vi "Image Browser Mod.vi"() -> ()   [LabVIEW 2016]
doc: "This example shows how to set up an image browser. An image browser is a concise representation of the images in your database represented as thumbnails on a page. You can use the Browser VIs in NI Vision to configure a browser, configure the selection of one or many images, add new images and remove images to and from a browser, replace an image, and get or set the selection status of an image."
uses:
  <vilib>/vision/NI_Vision_Development_Module.lvlib
panel:
  in  "Image folder":path=path "\\\\eden\\NHMFLDATA/Reference/Pressure/caliphotos/2018_04_12"
  out "Image":T1(plugin-control)
  in  "Stop":bool
  # "Overview: Demonstrates how to use the IMAQ Browser functions to display multiple thumbnail images in a single display. and allow the user to select images from the browser.\nRequirements: Vision Development Software.\nInstructions:\n1. Run the VI.\n2. Click on the images to select or unselect them."
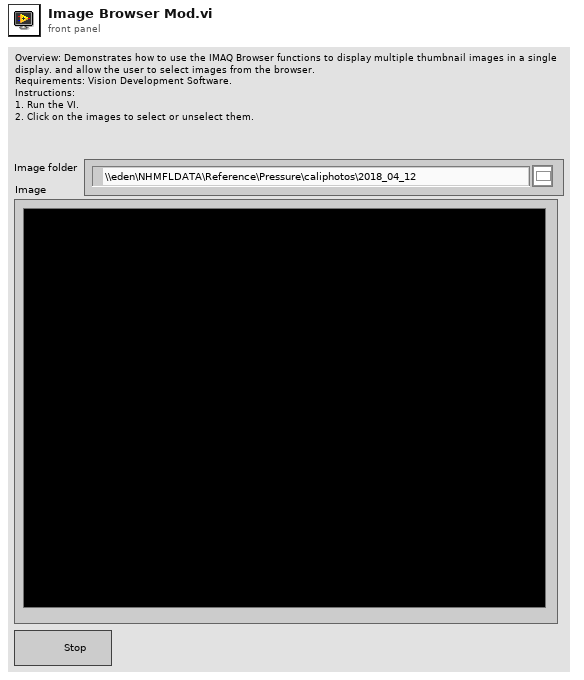
[diagram p1: front panel]
types:
  T1 = typedef "IMAQ Image.ctl" = refnum<image>
  T2 = cluster{"Browser Size":cluster{"X":i32, "Y":i32}, "Images per Line":i32, "Background Color":u32, "Frame Size":i32, "Frame Style":u16}
  T3 = typedef "Image Type" = u32
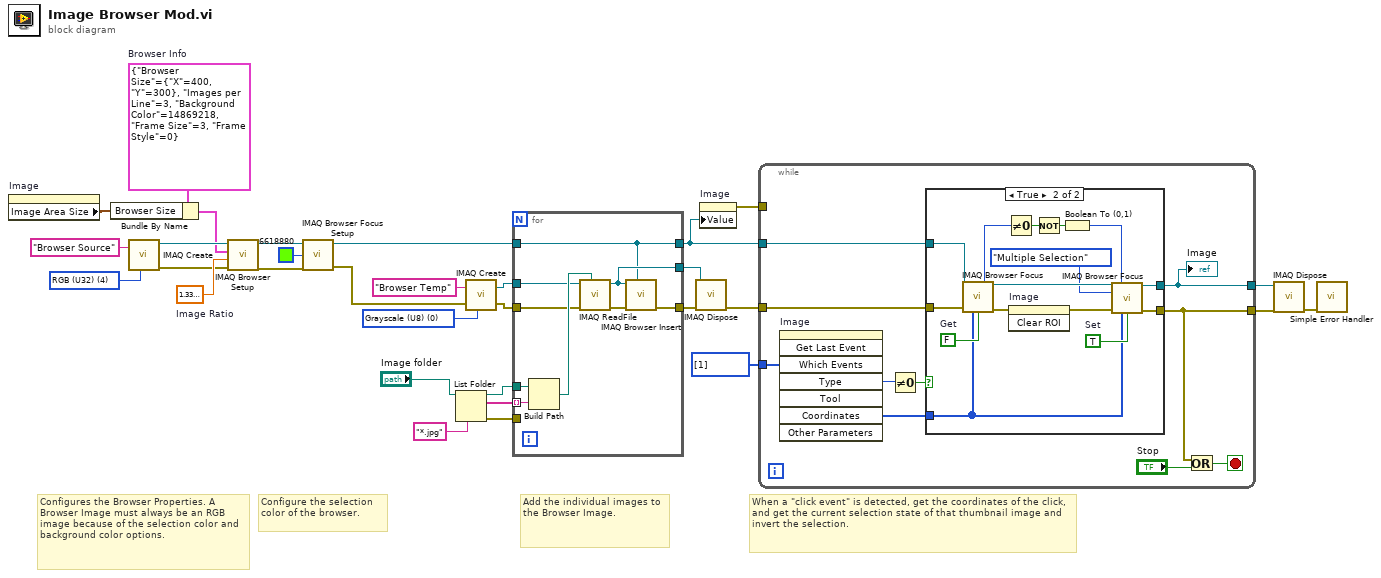
[diagram p0: block diagram]
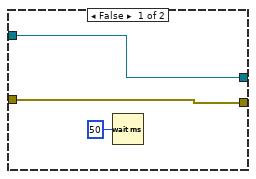
[diagram p2: hidden frame]
diagram:
  w18 = i32[] [1] items=["No Event"=0, "Click Event"=1, "Draw Event"=2, "Size Event"=4, "Scroll Event"=5, "Double Click Event"=8] ("Which Events")
  w31 = sgl 1.33  # Image Ratio
  w6 = T2 {"Browser Size"={"X"=400, "Y"=300}, "Images per Line"=3, "Background Color"=14869218, "Frame Size"=3, "Frame Style"=0}  # Browser Info
  w22 = T3 0 items=["Grayscale (U8)", "Grayscale (I16)", "Grayscale (SGL)", "Complex (CSG)", "RGB (U32)", "HSL (U32)", "RGB (U64)", "Grayscale (U16)"] ("Image Type")
  w24 = T3 4 items=["Grayscale (U8)", "Grayscale (I16)", "Grayscale (SGL)", "Complex (CSG)", "RGB (U32)", "HSL (U32)", "RGB (U64)", "Grayscale (U16)"] ("Image Type")
  # "When a \"click event\" is detected, get the coordinates of the click, and get the current selection state of that thumbnail image and invert the selection."
  # "Add the individual images to the Browser Image."
  # "Configure the selection color of the browser."
  # "Configures the Browser Properties. A Browser Image must always be an RGB image because of the selection color and background color options."
  n1 = property on="Image" class="ImageControl"() -> ("Image Area Size"=w5:cluster{"Width":u32, "Height":u32})  [unwired: 2 in, 2 out]
  n2 = Bundle By Name(cluster=w6, "Browser Size"=w5) -> (w4:T2)
  n3 = call "IMAQ Create"("Image Name"="Browser Source", "Image Type"=w24) -> ("New Image"=w26:T1, "error out"=w25:errorcluster)  [unwired: 3 in]
  n4 = call "IMAQ Browser Setup"("error in (no error)"=w25, "Image Ratio"=w31, "Browser Info"=w4, "Image In"=w26) -> ("error out"=w10:errorcluster, "Image Browser Out"=w11:T1)  [unwired: 2 out]
  n5 = call "IMAQ Browser Focus Setup"("error in (no error)"=w10, "Focus Color"=u32 6618880, "Image Browser In"=w11) -> ("error out"=w8:errorcluster, "Image Browser Out"=w9:T1)  [unwired: 1 in]
  n6 = List Folder(path="Image folder", pattern="*.jpg") -> (path out=w28:path, filenames=w27:string[], error out=w2:errorcluster)  [unwired: 2 in, 1 out]
  n7 = call "IMAQ Create"("Image Name"="Browser Temp", "Image Type"=w22, "error in (no error)"=w8) -> ("New Image"=w14:T1, "error out"=w30:errorcluster)  [unwired: 2 in]
  n8 = for {
    tunnel: w9 -> [w32]
    tunnel: w28 -> [w40]
    tunnel: w27 -> [w37] mode=indexing
    tunnel: w30 -> [w36]
    tunnel: [w35] -> w29
    tunnel: [w32] -> w19
    tunnel: w14 -> [w34]
    tunnel: [w33] -> w13
    tunnel: w2 -> [_]
    n9 = Build Path(base path=w40, name or relative path=w37) -> (appended path=w39:path)
    n10 = call "IMAQ ReadFile"("File Path"=w39, "error in (no error)"=w36, "Image"=w34) -> ("error out"=w38:errorcluster, "Image Out"=w33:T1)  [unwired: 4 in, 3 out]
    n11 = call "IMAQ Browser Insert"("Image Browser In"=w32, "error in (no error)"=w38, "Image to Add"=w33) -> ("error out"=w35:errorcluster)  [unwired: 4 in, 4 out]
  }
  n12 = call "IMAQ Dispose"("Image"=w13, "error in (no error)"=w29) -> ("error out"=w20:errorcluster)  [unwired: 4 in]
  n13 = property on="Image" class="ImageControl"("Value"=w19) -> (error out=w3:errorcluster)  [unwired: 2 in, 1 out]
  n14 = while {
    tunnel: w19 -> [w50]
    tunnel: w20 -> [w47]
    tunnel: w18 -> [w48]
    tunnel: [w45] -> w17
    tunnel: [w42] -> w16
    tunnel: w3 -> [_]
    stop <- w43 stop-if-true
    n15 = invoke on="Image" class="ImageControl" method="Get Last Event"("Which Events"=w48) -> ("Type"=w41:i32, "Coordinates"=w49:i32[])  [unwired: 7 in, 6 out]
    n16 = Not Equal To 0?(x=w41) -> (x != 0?=w46:bool)
    n17 = case shown="True" w46 {
      tunnel: w50 -> [w52 w68]
      tunnel: w49 -> [_ w59]
      tunnel: w47 -> [w53 w58]
      tunnel: [w53 w57] -> w45
      tunnel: [w52 w56] -> w42
      frame False {
        n18 = Wait (ms)(milliseconds to wait=u32 50) -> ()  [unwired: 1 out]
      }
      frame True {
        w66 = TRUE  # Set
        w67 = FALSE  # Get
        n19 = call "IMAQ Browser Focus"("Image Browser In"=w68, "error in (no error)"=w58, "Pixel Position"=w59, "Get/Set (Set)"=w67) -> ("State Out"=w63:enum16{"Not selected", "Selected"}, "Image Browser Out"=w65:T1, "error out"=w55:errorcluster)  [unwired: 6 in, 3 out]
        n20 = Not Equal To 0?(x=w63) -> (x != 0?=w61:bool)
        n21 = invoke on="Image" class="ImageControl" method="Clear ROI"(error in=w55) -> (error out=w54:errorcluster)  [unwired: 2 in, 2 out]
        n22 = Not(x=w61) -> (.not. x?=w60:bool)
        n23 = Boolean To (0,1)(Boolean=w60) -> (0, 1=w62:i16)
        n24 = call "IMAQ Browser Focus"("Image Browser In"=w65, "State In"=w62, "Selection Mode"=enum16{"Single Selection", "Multiple Selection"}."Multiple Selection", "error in (no error)"=w54, "Pixel Position"=w59, "Get/Set (Set)"=w66) -> ("Image Browser Out"=w56:T1, "error out"=w57:errorcluster)  [unwired: 4 in, 4 out]
      }
    }
    "Image" <- w42
    n25 = Or(x=w45, y="Stop") -> (x .or. y?=w43:bool)
  }
  n26 = call "IMAQ Dispose"("Image"=w16, "error in (no error)"=w17) -> ("error out"=w15:errorcluster)  [unwired: 4 in]
  n27 = call <vilib>:"Simple Error Handler.vi"("error in (no error)"=w15) -> ()  [unwired: 4 in, 5 out]
